vi "Get (U32).vi"(8 "error in":errorcluster, 11 "Value in":refnum<class "Value.lvclass">) -> (0 "error out":errorcluster, 1 "Is Defined?":bool, 2 "Value":u32, 3 "Value out":refnum<class "Value.lvclass">)   [LabVIEW 2019, in "Electronic Datasheet.lvlib" / "Value.lvclass"]
uses:
  Value.lvclass
  Value.lvclass/Value.ctl
  Electronic Datasheet.lvlib
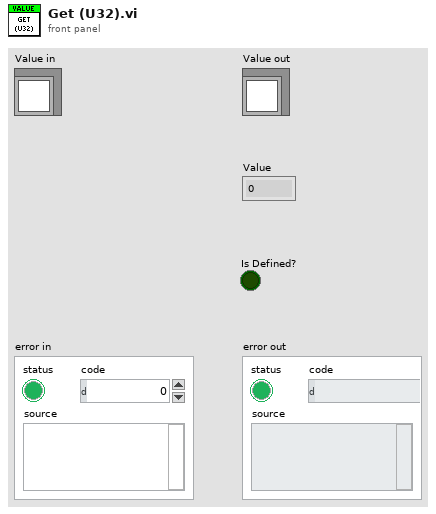
[diagram p1: front panel]
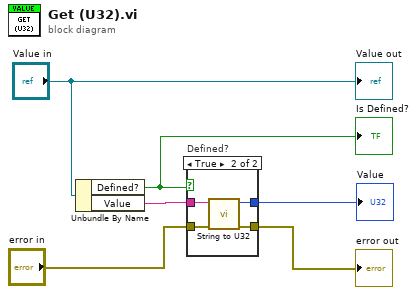
[diagram p0: block diagram]
diagram:
  n1 = Unbundle By Name("Value in") -> ("Defined?"=w1:bool, "Value"=w5:string)
  "Is Defined?" <- w1
  n2 = case "Defined?" shown="True" w1 {
    tunnel: w5 -> [_ w11]
    tunnel: [_ w10] -> w4
    tunnel: "error in" -> [w7 w9]
    tunnel: [w7 w8] -> w2
    frame False {
    }
    frame True {
      n3 = call "String to U32.vi"("error in"=w9, "Integer String"=w11) -> ("error out"=w8:errorcluster, "U32"=w10:u32)  [unwired: 8 in]
    }
  }
  "Value" <- w4
  "error out" <- w2
  "Value out" <- "Value in"
